vi "PE Open.vi"(8 "error in (no error)":errorcluster, 10 "name":string, 11 "peHandle":u32) -> (0 "error out":errorcluster)   [LabVIEW 2017, in "PE_Filter_SDK.lvlib"]
doc: "PEFILTERSDK_API PE_STATUS PE_Open(PE_HANDLE peHandle, const char* name);"
uses:
  PE_Filter_SDK.lvlib
  PE_Filter_SDK.dll
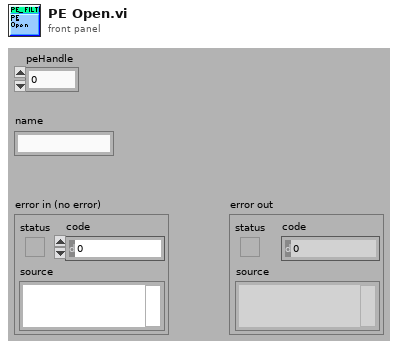
[diagram p1: front panel]
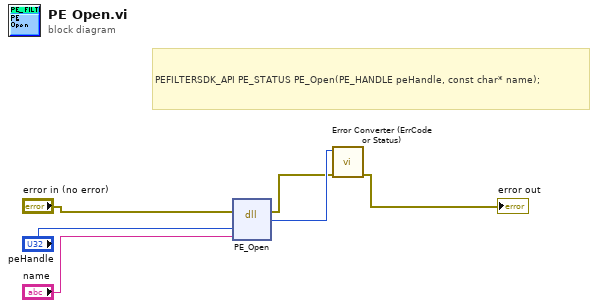
[diagram p0: block diagram]
diagram:
  # "PEFILTERSDK_API PE_STATUS PE_Open(PE_HANDLE peHandle, const char* name);"
  n1 = dll-call lib="PE_Filter_SDK.*" fn="PE_Open"(error in="error in (no error)", "peHandle"="peHandle", "name"="name") -> (error out=w2:errorcluster, w3:u32)  [unwired: 4 in, 1 out]
  n2 = call "Error Converter (ErrCode or Status).vi"("error in (no error)"=w2, "error code"=w3) -> ("error out"=→"error out":errorcluster)  [unwired: 9 in]
